vi "Random Unused Color.vi"(11 "existing colors":u32[](array[colorbox])) -> (3 "new color":u32(colorbox))   [LabVIEW 2017, in "NI_Robotics_Control Utilities.lvlib"]
uses:
  <vilib>/robotics/Controls/Utilities/NI_Robotics_Control Utilities.lvlib
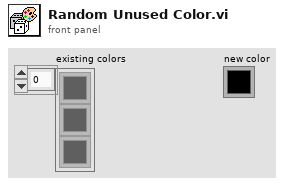
[diagram p1: front panel]
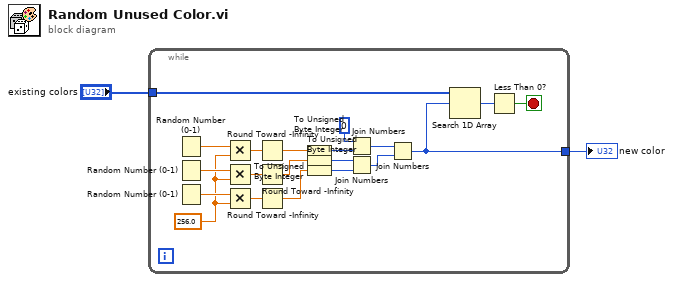
[diagram p0: block diagram]
diagram:
  n1 = while {
    tunnel: "existing colors" -> [w12]
    tunnel: [w11] -> w1
    stop <- w9 stop-if-true
    w15 = 256.0 ("y")
    n2 = Random Number (0-1)() -> (number: 0 to 1=w22:dbl)
    n3 = Random Number (0-1)() -> (number: 0 to 1=w17:dbl)
    n4 = Random Number (0-1)() -> (number: 0 to 1=w16:dbl)
    n5 = Multiply(x=w22, y=w15) -> (x*y=w21:dbl)
    n6 = Multiply(x=w17, y=w15) -> (x*y=w19:dbl)
    n7 = Multiply(x=w16, y=w15) -> (x*y=w18:dbl)
    n8 = Round Toward -Infinity(1:w21) -> (0:w20:dbl)
    n9 = Round Toward -Infinity(1:w19) -> (0:w14:dbl)
    n10 = Round Toward -Infinity(1:w18) -> (0:w13:dbl)
    n11 = To Unsigned Byte Integer(number=w20) -> (unsigned 8bit integer=w8:u8)
    n12 = To Unsigned Byte Integer(number=w14) -> (unsigned 8bit integer=w7:u8)
    n13 = To Unsigned Byte Integer(number=w13) -> (unsigned 8bit integer=w6:u8)
    n14 = Join Numbers(hi=u8 0, lo=w8) -> ((hi.lo)=w4:u16)
    n15 = Join Numbers(hi=w7, lo=w6) -> ((hi.lo)=w5:u16)
    n16 = Join Numbers(hi=w4, lo=w5) -> ((hi.lo)=w11:u32)
    n17 = Search 1D Array(1D array=w12, element=w11) -> (index of element=w10:i32)  [unwired: 1 in]
    n18 = Less Than 0?(x=w10) -> (x < 0?=w9:bool)
  }
  "new color" <- w1
